vi "Test Code.vi"() -> ()   [LabVIEW 2011]
panel:
  out "x*y":dbl
  in  "Tire Diameter":dbl
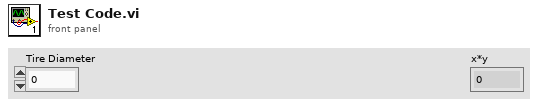
[diagram p1: front panel]
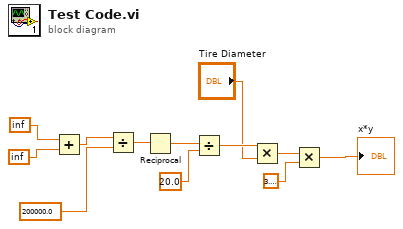
[diagram p0: block diagram]
diagram:
  n1 = Add(x=inf, y=inf) -> (x+y=w10:dbl)
  n2 = Divide(x=w10, y=200000.0) -> (x/y=w8:dbl)
  n3 = Reciprocal(x=w8) -> (1/x=w7:dbl)
  n4 = Divide(x=w7, y=20.0) -> (x/y=w5:dbl)
  n5 = Multiply(x=w5, y="Tire Diameter") -> (x*y=w3:dbl)
  n6 = Multiply(x=w3, y=3.141592653589793) -> (x*y=→"x*y":dbl)
